vi "Joysticks.vi"(0 "SRE Enum":enum16{"Start", "Run", "End"}(ring)) -> (7 "Left joy":dbl, 8 "Right joy":dbl)   [LabVIEW 2014]
uses:
  <vilib>/Rock Robotics/WPI/Joystick/WPI_JoystickDeviceEnum.ctl
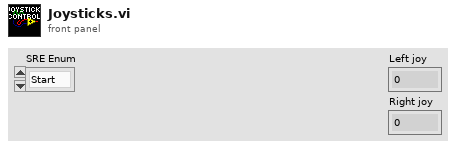
[diagram p1: front panel]
types:
  T1 = typedef "WPI_JoystickDeviceEnum.ctl" = enum16{"USB 0", "USB 1", "USB 2", "USB 3", "USB 4", "USB 5"}
  T2 = typedef "WPI_JoystickDevRef.ctl" = cluster{"Device":T1}
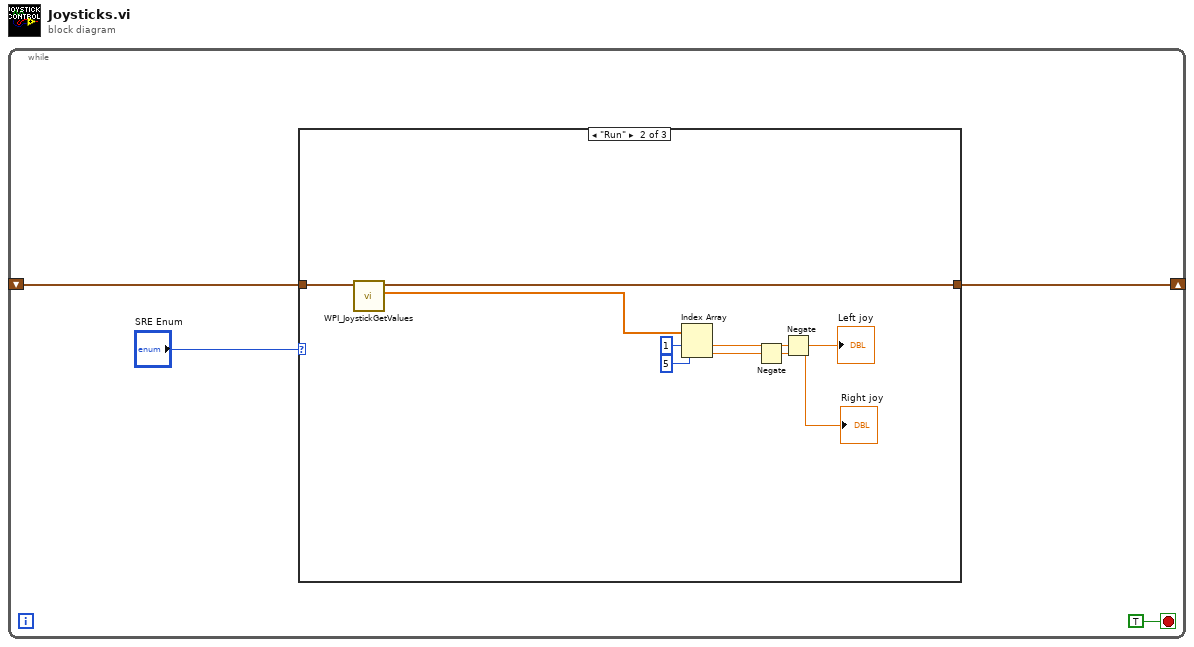
[diagram p0: block diagram]
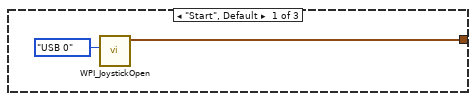
[diagram p2: hidden frame]
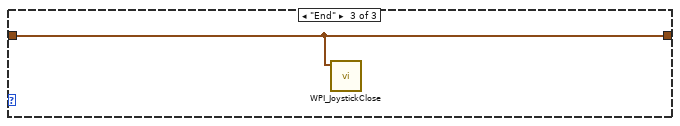
[diagram p3: hidden frame]
diagram:
  n1 = while {
    shift-right: [w3] -> _
    shift-left: _ -> [w2]
    stop <- TRUE stop-if-true
    n2 = case shown="\"Run\"" "SRE Enum" {
      tunnel: [w6 w15 w16] -> w3
      tunnel: w2 -> [_ w14 w16]
      frame "Start", Default {
        n3 = call <vilib>:"WPI_JoystickOpen.vi"("JoystickDevice"=WPI_JoystickDeviceEnum."USB 0") -> ("JoystickDevRef"=w6:T2)  [unwired: 10 in]
      }
      frame "Run" {
        n4 = call <vilib>:"WPI_JoystickGetValues.vi"("JoystickDevRef"=w14) -> ("Axes"=w9:dbl[], "JoystickDevRef"=w15:T2)  [unwired: 6 in, 3 out]
        n5 = Index Array(array=w9, index #1=1 ("index"), index #2=5 ("index")) -> (element #1=w11:dbl, element #2=w10:dbl)
        n6 = Negate(x=w10) -> (-x=→"Right joy":dbl)
        n7 = Negate(x=w11) -> (-x=→"Left joy":dbl)
      }
      frame "End" {
        n8 = call <vilib>:"WPI_JoystickClose.vi"("JoystickDevRef"=w16) -> ()  [unwired: 11 in]
      }
    }
  }
